vi "getNsetVIinfo.vi"(8 "Resave if required":bool=TRUE, 9 "Disable Automatic Error Handling":bool=TRUE, 10 "Remove Compiled Code":bool=TRUE, 11 "path":path) -> (0 "values":string[](array[string]), 1 "titles":string[](array[string]), 4 "Execution:State":T3(ring))   [LabVIEW 2022 SP3]
panel:
  out "VI:Save:State":string
  out "Auto:Error:Handling?":string
  out "Contains:Compiled:Code?":string
  out "error out":errorcluster
  out "VI:Total:Size":u32
  out "LabVIEW:Revision:Number":u32
  out "Number:of:subVIs":i32
  out "Execution:Priority":T1(ring)
  out "Execution:Thread":T2(ring)
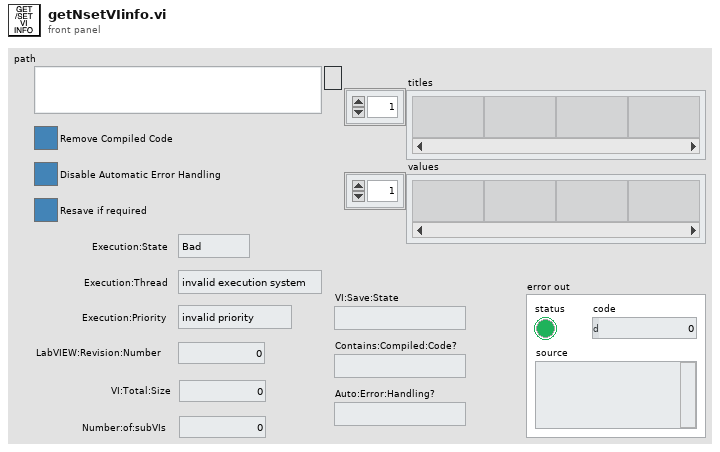
[diagram p1: front panel]
types:
  T1 = enum32{"invalid priority", "background priority", "normal priority", "above normal priority", "high priority", "time critical priority", "subroutine"}
  T2 = enum32{"invalid execution system", "user interface", "standard", "instrument i/o", "data acquisition", "other 1", "other 2", "same as caller"}
  T3 = enum32{"Bad", "Idle", "Run top level", "Running"}
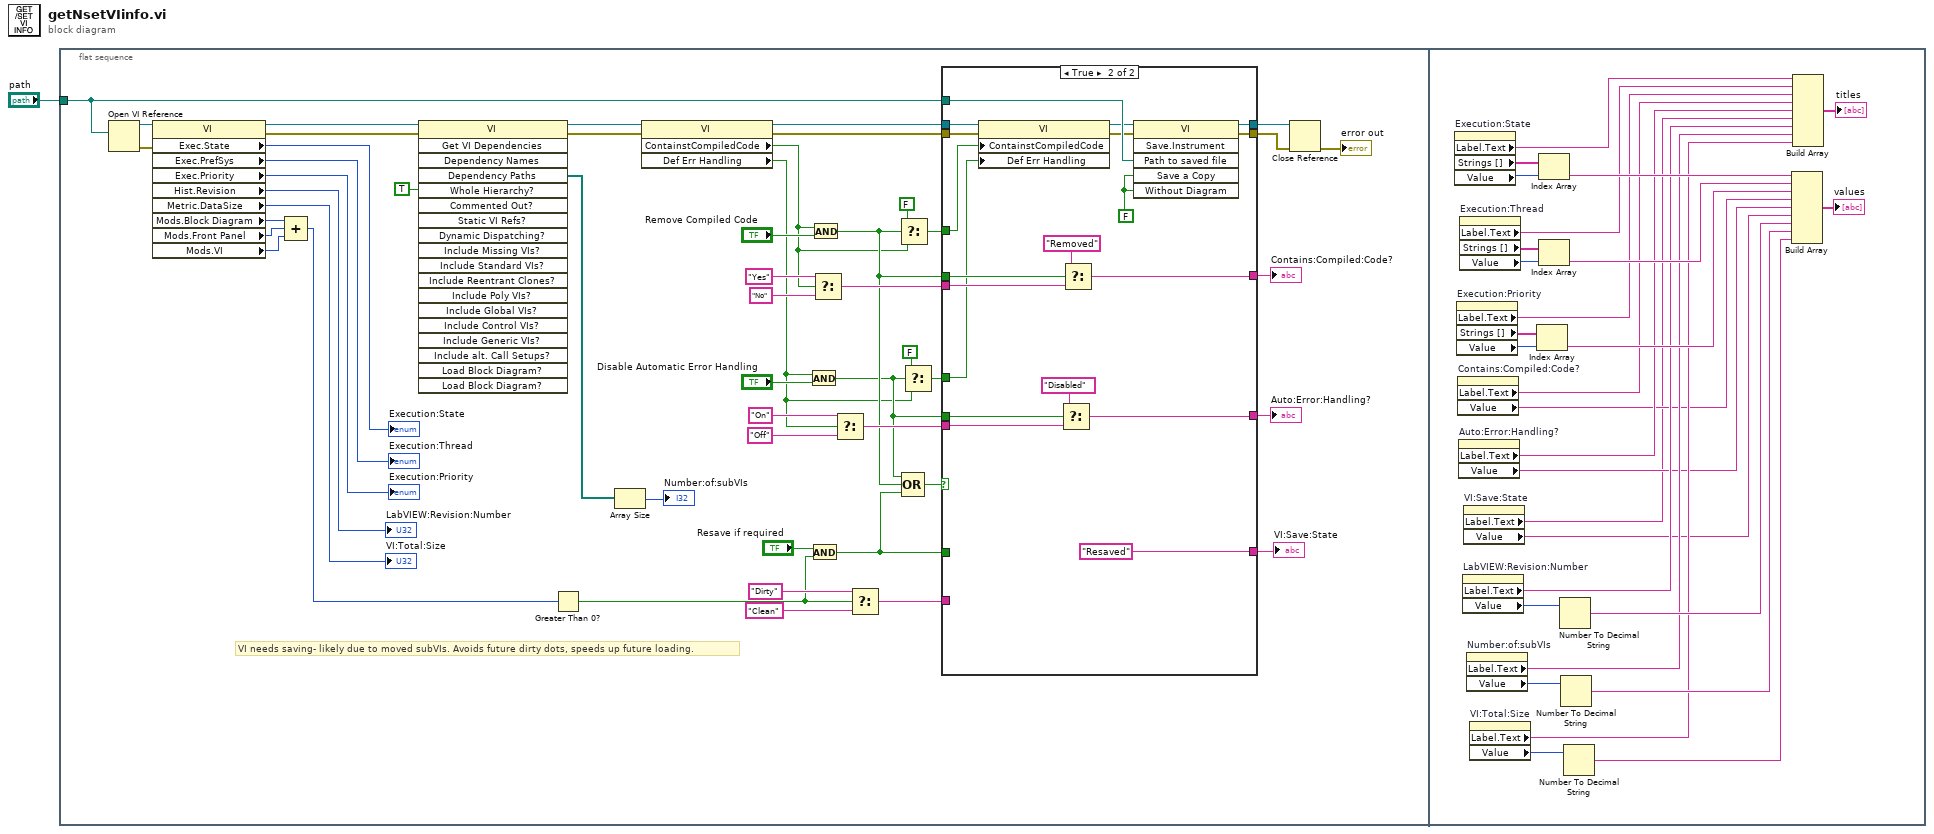
[diagram p0: block diagram]
diagram:
  n1 = flat-sequence {
    tunnel: "path" -> [w45]
    frame #0 {
      # "VI needs saving- likely due to moved subVIs. Avoids future dirty dots, speeds up future loading."
      n2 = Open VI Reference(vi path=w45) -> (vi reference=w16:refnum<vi>, error out=w15:errorcluster)  [unwired: 5 in]
      n3 = property class="VI"(reference=w16, error in=w15) -> (reference out=w29:refnum<vi>, error out=w28:errorcluster, "Exec.State"=→"Execution:State":T3, "Exec.PrefSys"=→"Execution:Thread":T2, "Exec.Priority"=→"Execution:Priority":T1, "Hist.Revision"=→"LabVIEW:Revision:Number":u32, "Metric.DataSize"=→"VI:Total:Size":u32, "Mods.Block Diagram"=w12:u32, "Mods.Front Panel"=w11:u32, "Mods.VI"=w10:u64)
      n4 = Compound Arithmetic op=ADD(w12, w11, w10) -> (w9:u64)
      n5 = invoke class="VI" method="Get VI Dependencies"(reference=w29, error in=w28, "Whole Hierarchy?"=TRUE) -> (reference out=w18:refnum<vi>, error out=w17:errorcluster, "Dependency Paths"=w31:path[])  [unwired: 16 in, 16 out]
      n6 = Greater Than 0?(x=w9) -> (x > 0?=w5:bool)
      n7 = Array Size(array=w31) -> (size(s)=→"Number:of:subVIs":i32)
      n8 = property class="VI"(reference=w18, error in=w17) -> (reference out=w43:refnum<vi>, error out=w42:errorcluster, "ContainstCompiledCode"=w25:bool, "Def Err Handling"=w22:bool)
      n9 = And(x=w22, y="Disable Automatic Error Handling") -> (x .and. y?=w24:bool)
      n10 = And(x="Resave if required", y=w5) -> (x .and. y?=w3:bool)
      n11 = And(x=w25, y="Remove Compiled Code") -> (x .and. y?=w27:bool)
      n12 = Select(t="Yes", s=w25, f="No") -> (s? t:f=w39:string)
      n13 = Select(t="On", s=w22, f="Off") -> (s? t:f=w35:string)
      n14 = Select(t="Dirty", s=w5, f="Clean") -> (s? t:f=w4:string)
      n15 = Select(t=FALSE, s=w27, f=w25) -> (s? t:f=w23:bool)
      n16 = Compound Arithmetic op=OR(w24, w27, w3) -> (w44:bool)
      n17 = Select(t=FALSE, s=w24, f=w22) -> (s? t:f=w20:bool)
      n18 = case shown="True" w44 {
        tunnel: w43 -> [w56 w71]
        tunnel: w42 -> [w55 w68]
        tunnel: [w56 w75] -> w14
        tunnel: [w55 w74] -> w13
        tunnel: w45 -> [_ w72]
        tunnel: w27 -> [_ w67]
        tunnel: w24 -> [_ w65]
        tunnel: w39 -> [w54 w63]
        tunnel: w35 -> [w53 w62]
        tunnel: [w54 w61] -> w34
        tunnel: [w53 w60] -> w33
        tunnel: w23 -> [_ w59]
        tunnel: w20 -> [_ w58]
        tunnel: w4 -> [w52 _]
        tunnel: w3 -> [_ _]
        tunnel: [w52 "Resaved"] -> w2
        frame False {
        }
        frame True {
          w73 = FALSE ("Save a Copy")
          n19 = property class="VI"(reference=w71, error in=w68, "ContainstCompiledCode"=w59, "Def Err Handling"=w58) -> (reference out=w70:refnum<vi>, error out=w69:errorcluster)
          n20 = Select(t="Disabled", s=w65, f=w62) -> (s? t:f=w60:string)
          n21 = Select(t="Removed", s=w67, f=w63) -> (s? t:f=w61:string)
          n22 = invoke class="VI" method="Save.Instrument"(reference=w70, error in=w69, "Path to saved file"=w72, "Save a Copy"=w73, "Without Diagram"=w73) -> (reference out=w75:refnum<vi>, error out=w74:errorcluster)  [unwired: 1 in, 4 out]
        }
      }
      "Contains:Compiled:Code?" <- w34
      "Auto:Error:Handling?" <- w33
      "VI:Save:State" <- w2
      n23 = Close Reference(reference=w14, error in (no error)=w13) -> (error out=→"error out":errorcluster)
    }
    frame #1 {
      n24 = property on="Execution:State" class="Enum (strict)"() -> ("Label.Text"=w86:string, "Strings []"=w83:string[], "Value"=w95:T3)  [unwired: 2 in, 2 out]
      n25 = property on="Execution:Priority" class="Enum (strict)"() -> ("Label.Text"=w88:string, "Strings []"=w85:string[], "Value"=w97:T1)  [unwired: 2 in, 2 out]
      n26 = property on="Contains:Compiled:Code?" class="Str"() -> ("Label.Text"=w89:string, "Value"=w79:string)  [unwired: 2 in, 2 out]
      n27 = property on="Auto:Error:Handling?" class="Str"() -> ("Label.Text"=w90:string, "Value"=w78:string)  [unwired: 2 in, 2 out]
      n28 = property on="Execution:Thread" class="Enum (strict)"() -> ("Label.Text"=w87:string, "Strings []"=w84:string[], "Value"=w96:T2)  [unwired: 2 in, 2 out]
      n29 = property on="LabVIEW:Revision:Number" class="DigNum (strict)"() -> ("Label.Text"=w91:string, "Value"=w94:u32)  [unwired: 2 in, 2 out]
      n30 = property on="VI:Save:State" class="Str"() -> ("Label.Text"=w77:string, "Value"=w76:string)  [unwired: 2 in, 2 out]
      n31 = property on="Number:of:subVIs" class="DigNum (strict)"() -> ("Label.Text"=w92:string, "Value"=w93:i32)  [unwired: 2 in, 2 out]
      n32 = property on="VI:Total:Size" class="DigNum (strict)"() -> ("Label.Text"=w81:string, "Value"=w82:u32)  [unwired: 2 in, 2 out]
      n33 = Index Array(array=w85, index=w97) -> (element=w100:string)
      n34 = Index Array(array=w83, index=w95) -> (element=w98:string)
      n35 = Index Array(array=w84, index=w96) -> (element=w99:string)
      n36 = Number To Decimal String(number=w94) -> (decimal integer string=w101:string)  [unwired: 1 in]
      n37 = Number To Decimal String(number=w93) -> (decimal integer string=w102:string)  [unwired: 1 in]
      n38 = Number To Decimal String(number=w82) -> (decimal integer string=w80:string)  [unwired: 1 in]
      n39 = Build Array(w98, w99, w100, w79, w78, w76, w101, w102, w80) -> (→"values":string[])
      n40 = Build Array(w86, w87, w88, w89, w90, w77, w91, w92, w81) -> (→"titles":string[])
    }
  }
